vi "XY Graph Init.vi"(4 "Graph Tool Panels Visibility":T1={"Scale Legend Vis"=TRUE, "X-Scrollbar Vis"=FALSE, "Cursor Panel Vis"=FALSE, "Graph Palette Vis"=TRUE}, 6 "Max Legend Size (8)":i32=8, 8 "Error In":errorcluster, 9 "Plots to Skip (none)":i32[](array[numeric]), 10 "Metadata Type":variant, 11 "XYGraph in":T2) -> (0 "Error Out":errorcluster)   [LabVIEW 2021, in "XY Graph Add-Ons.lvlib"]
doc: "Clears Plot Names and restores their visibility"
uses:
  XY Graph Add-Ons.lvlib
  XY Graph Refnum.ctl
  XY Graph Tool Panels Visibility.ctl
  XY Graph Property Tag List.ctl
  XY Graph Set Max Legend Size.vi
  XY Graph Set Plots to Preserve.vi
  XY Graph Set TipStrip String.vi
  XY Graph Set TipStrip Visible.vi
  XY Graph Set Tool Panels Visibility.vi
  XY Graph Set Plots Metadata.vi
  Graphs.lvlib
  Error/Error.lvlib
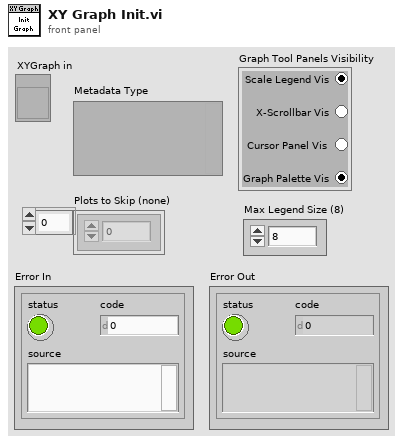
[diagram p1: front panel]
types:
  T1 = typedef "XY Graph Add-Ons.lvlib/XY Graph Tool Panels Visibility.ctl" = cluster{"Scale Legend Vis":bool, "X-Scrollbar Vis":bool, "Cursor Panel Vis":bool, "Graph Palette Vis":bool}
  T2 = typedef "XY Graph Add-Ons.lvlib/XY Graph Refnum.ctl" = refnum<vi>
  T3 = typedef "XY Graph Add-Ons.lvlib/XY Graph Property Tag List.ctl" = enum16{"Max Legend Size", "Preserved Plots", "XScales.GridColors", "YScales.GridColors", "TipStrip String", "TipStrip Visible", "Tool Panels Visibility", "Plot Metadata"}
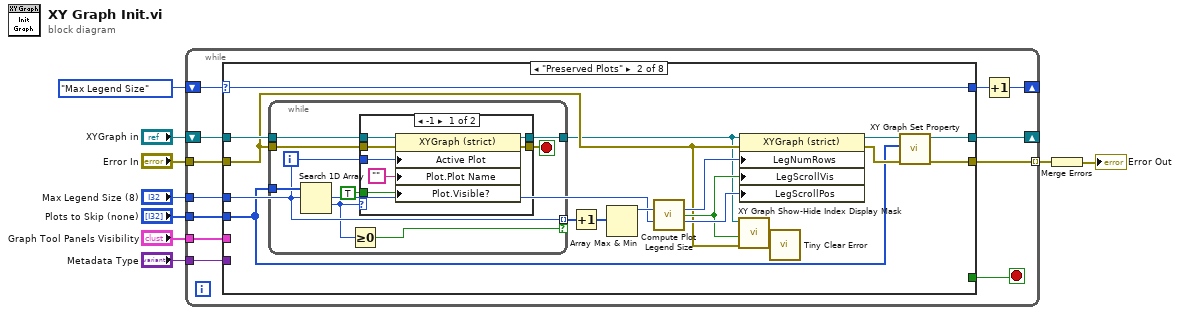
[diagram p0: block diagram]
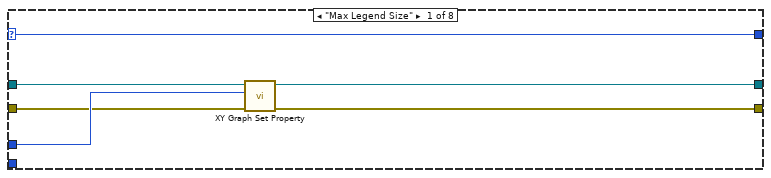
[diagram p2: hidden frame]
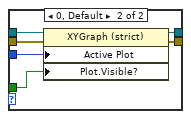
[diagram p3: hidden frame]
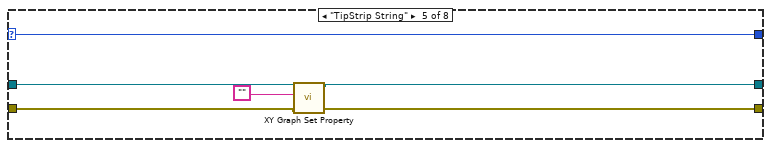
[diagram p6: hidden frame]
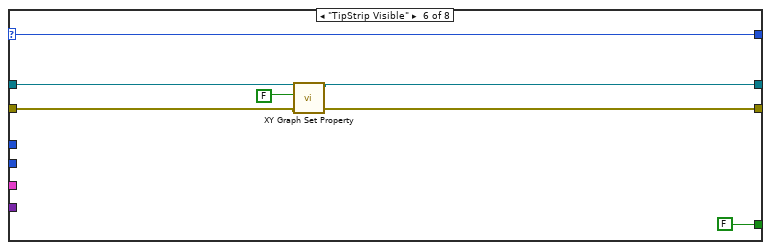
[diagram p7: hidden frame]
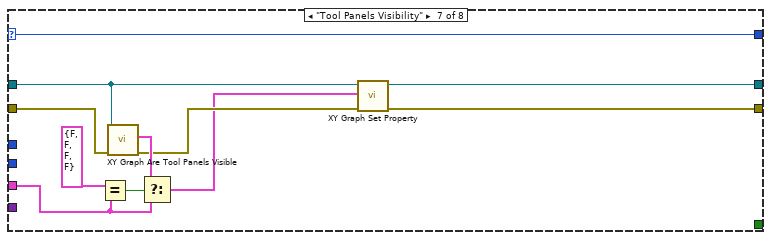
[diagram p8: hidden frame]
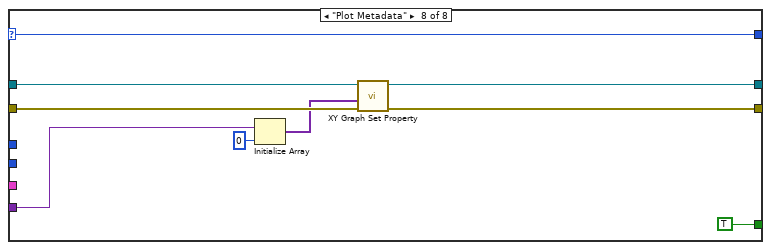
[diagram p9: hidden frame]
diagram:
  n1 = while {
    tunnel: "Error In" -> [w20]
    tunnel: "Plots to Skip (none)" -> [w19]
    tunnel: "Max Legend Size (8)" -> [w18]
    shift-right: [w15] -> _
    shift-left: XY_Graph_Property_Tag_List."Max Legend Size" ("XY Graph Property Tag") -> [w17]
    shift-right: [w13] -> _
    shift-left: "XYGraph in" -> [w21]
    tunnel: [w12] -> w4 mode=indexing
    tunnel: "Graph Tool Panels Visibility" -> [w11]
    tunnel: "Metadata Type" -> [w10]
    stop <- w14 stop-if-true
    n2 = case shown="\"Preserved Plots\"" w17 {
      selector: w17 -> [w27 w37 w68 w71 w78 w85 w96 w105]
      tunnel: w21 -> [w25 w44 w69 w72 w77 w84 w92 w101]
      tunnel: w20 -> [w23 w29 w67 w70 w76 w83 w89 w100]
      tunnel: w19 -> [_ w32 _ _ _ _ _ _]
      tunnel: w18 -> [w26 w38 _ _ _ _ _ _]
      tunnel: [w27 w37 w68 w71 w78 w85 w96 w105] -> w16
      tunnel: [_ _ _ _ _ FALSE _ TRUE] -> w14
      tunnel: [w24 w33 w69 w72 w75 w82 w95 w104] -> w13
      tunnel: [w22 w34 w67 w70 w74 w81 w94 w103] -> w12
      tunnel: w11 -> [_ _ _ _ _ _ w86 _]
      tunnel: w10 -> [_ _ _ _ _ _ _ w99]
      frame "Max Legend Size" {
        n3 = call-poly "XY Graph Set Property.vi"("error in (no error)"=w23, "Max Legend Size"=w26, "XY Graph Refnum"=w25) -> ("error out"=w22:errorcluster, "XY Graph Refnum (dup)"=w24:T2)  [unwired: 7 in]
      }
      frame "Preserved Plots" {
        n4 = while {
          tunnel: w44 -> [w53]
          tunnel: w29 -> [w51]
          tunnel: w32 -> [w50]
          tunnel: [w48] -> w43 mode=indexing if=w46
          tunnel: [w45] -> w28
          i -> [w48]
          stop <- w52 stop-if-true
          n5 = Search 1D Array(1D array=w50, element=w48) -> (index of element=w47:i32)  [unwired: 1 in]
          n6 = Greater Or Equal To 0?(x=w47) -> (x >= 0?=w46:bool)
          n7 = case shown="-1" w47 {
            tunnel: w53 -> [w60 w64]
            tunnel: [w59 w63] -> w52
            tunnel: w51 -> [w58 w65]
            tunnel: w48 -> [w57 w66]
            tunnel: TRUE ("Plot.Visible") -> [w55 w62]
            tunnel: [w54 w61] -> w45
            frame -1 {
              n8 = property class="XYGraph (strict)"(reference=w60, error in=w58, "Active Plot"=w57, "Plot.Plot Name"="", "Plot.Visible?"=w55) -> (reference out=w54:T2, error out=w59:errorcluster)
            }
            frame 0, Default {
              n9 = property class="XYGraph (strict)"(reference=w64, error in=w65, "Active Plot"=w66, "Plot.Visible?"=w62) -> (reference out=w61:T2, error out=w63:errorcluster)
            }
          }
        }
        n10 = Increment(x=w43) -> (x+1=w42:i32[])
        n11 = Array Max & Min(array=w42) -> (max value=w41:i32)  [unwired: 3 out]
        n12 = call "Compute Plot Legend Size.vi"("# Plots"=w41, "Max Legend Size"=w38) -> ("LegNumRows"=w40:u32, "LegScrollVis"=w30:bool, "LegScrollPos"=w39:u32)  [unwired: 11 in]
        n13 = call "XY Graph Show-Hide Index Display Mask.vi"("error in (no error)"=w29, "Show(T)/Hide(F)"=w30, "XYGraph Ref"=w28) -> ("error out"=w31:errorcluster)  [unwired: 7 in, 1 out]
        n14 = property class="XYGraph (strict)"(reference=w28, error in=w29, "LegNumRows"=w40, "LegScrollVis"=w30, "LegScrollPos"=w39) -> (reference out=w36:T2, error out=w35:errorcluster)
        n15 = call "Tiny Clear Error.vi"("Error In"=w31) -> ()  [unwired: 8 in, 1 out]
        n16 = call-poly "XY Graph Set Property.vi"("error in (no error)"=w35, "Plots to Preserve"=w32, "XY Graph Refnum"=w36) -> ("error out"=w34:errorcluster, "XY Graph Refnum (dup)"=w33:T2)  [unwired: 7 in]
      }
      frame "XScales.GridColors" {
      }
      frame "YScales.GridColors" {
      }
      frame "TipStrip String" {
        n17 = call-poly "XY Graph Set Property.vi"("error in (no error)"=w76, "TipStrip String"="", "XY Graph Refnum"=w77) -> ("error out"=w74:errorcluster, "XY Graph Refnum (dup)"=w75:T2)  [unwired: 6 in, 1 out]
      }
      frame "TipStrip Visible" {
        n18 = call-poly "XY Graph Set Property.vi"("error in (no error)"=w83, "TipStrip Visible"=FALSE, "XY Graph Refnum"=w84) -> ("error out"=w81:errorcluster, "XY Graph Refnum (dup)"=w82:T2)  [unwired: 6 in, 1 out]
      }
      frame "Tool Panels Visibility" {
        n19 = Equal?(x=T1 {"Scale Legend Vis"=FALSE, "X-Scrollbar Vis"=FALSE, "Cursor Panel Vis"=FALSE, "Graph Palette Vis"=FALSE} ("y"), y=w86) -> (x = y?=w93:bool)
        n20 = call "XY Graph Are Tool Panels Visible.vi"("Error In"=w89, "XY Graph Ref"=w92) -> ("Error Out"=w90:errorcluster, "Graph Tool Panels Visibility"=w91:T1)  [unwired: 6 in, 2 out]
        n21 = Select(t=w91, s=w93, f=w86) -> (s? t:f=w88:T1)
        n22 = call-poly "XY Graph Set Property.vi"("error in (no error)"=w90, "Graph Tool Panels Visibility"=w88, "XYGraph in"=w92) -> ("error out"=w94:errorcluster, "XYGraph out"=w95:T2)  [unwired: 7 in]
      }
      frame "Plot Metadata" {
        n23 = Initialize Array(w99, 0 ("dimension size")) -> (w97:variant[])
        n24 = call-poly "XY Graph Set Property.vi"("error in (no error)"=w100, "Plots Metadata"=w97, "XY Graph Refnum"=w101) -> ("error out"=w103:errorcluster, "XY Graph Refnum (dup)"=w104:T2)  [unwired: 7 in]
      }
    }
    n25 = Increment(x=w16) -> (x+1=w15:T3)
  }
  n26 = Merge Errors(w4) -> (→"Error Out":errorcluster)
